vi "Lab Panel V4.90.vi"() -> ()   [LabVIEW 2013] (continued)
                              tunnel: [w5375 0] -> w5370
                              tunnel: w5371 -> [w5375 _]
                              tunnel: w5372 -> [_ w5376]
                              frame False {
                              }
                              frame True {
                                n2891 = Concatenate Strings("LA02-2 ", w5376) -> (w5379:string)
                                n2892 = One Button Dialog(message=w5379) -> ()  [unwired: 1 in, 1 out]
                              }
                            }
                          }
                          frame #4 {
                            n2893 = Greater?(x=w5381, y=w5384) -> (0:w5383:bool)
                            n2894 = case shown="True" w5383 {
                              tunnel: [w5385 0] -> w5380
                              tunnel: w5381 -> [w5385 _]
                              tunnel: w5382 -> [_ w5386]
                              frame False {
                              }
                              frame True {
                                n2895 = Concatenate Strings("LA03-1 ", w5386) -> (w5389:string)
                                n2896 = One Button Dialog(message=w5389) -> ()  [unwired: 1 in, 1 out]
                              }
                            }
                          }
                          frame #5 {
                            n2897 = Greater?(x=w5390, y=w5394) -> (0:w5393:bool)
                            n2898 = case shown="True" w5393 {
                              tunnel: [w5395 0] -> w5391
                              tunnel: w5390 -> [w5395 _]
                              tunnel: w5392 -> [_ w5396]
                              frame False {
                              }
                              frame True {
                                n2899 = Concatenate Strings("LA03-2 ", w5396) -> (w5399:string)
                                n2900 = One Button Dialog(message=w5399) -> ()  [unwired: 1 in, 1 out]
                              }
                            }
                          }
                          frame #6 {
                            n2901 = Greater?(x=w5401, y=w5404) -> (0:w5403:bool)
                            n2902 = case shown="True" w5403 {
                              tunnel: [w5405 0] -> w5400
                              tunnel: w5401 -> [w5405 _]
                              tunnel: w5402 -> [_ w5406]
                              frame False {
                              }
                              frame True {
                                n2903 = Concatenate Strings("LA04-1 ", w5406) -> (w5409:string)
                                n2904 = One Button Dialog(message=w5409) -> ()  [unwired: 1 in, 1 out]
                              }
                            }
                          }
                          frame #7 {
                            n2905 = Greater?(x=w5411, y=w5414) -> (0:w5413:bool)
                            n2906 = case shown="True" w5413 {
                              tunnel: [w5415 0] -> w5410
                              tunnel: w5411 -> [w5415 _]
                              tunnel: w5412 -> [_ w5416]
                              frame False {
                              }
                              frame True {
                                n2907 = Concatenate Strings("LA04-2 ", w5416) -> (w5419:string)
                                n2908 = One Button Dialog(message=w5419) -> ()  [unwired: 1 in, 1 out]
                              }
                            }
                          }
                          frame #8 {
                            n2909 = Greater?(x=w5421, y=w5424) -> (0:w5423:bool)
                            n2910 = case shown="True" w5423 {
                              tunnel: [w5425 0] -> w5420
                              tunnel: w5421 -> [w5425 _]
                              tunnel: w5422 -> [_ w5426]
                              frame False {
                              }
                              frame True {
                                n2911 = Concatenate Strings("LA05-1 ", w5426) -> (w5429:string)
                                n2912 = One Button Dialog(message=w5429) -> ()  [unwired: 1 in, 1 out]
                              }
                            }
                          }
                          frame #9 {
                            n2913 = Greater?(x=w5431, y=w5434) -> (0:w5433:bool)
                            n2914 = case shown="True" w5433 {
                              tunnel: [w5435 0] -> w5430
                              tunnel: w5431 -> [w5435 _]
                              tunnel: w5432 -> [_ w5436]
                              frame False {
                              }
                              frame True {
                                n2915 = Concatenate Strings("LA05-2 ", w5436) -> (w5439:string)
                                n2916 = One Button Dialog(message=w5439) -> ()  [unwired: 1 in, 1 out]
                              }
                            }
                          }
                        }
                        n2917 = Bundle By Name(cluster=w5338, "LAB01-1"=w5336, "LAB01-2"=w5334, "LAB02-1"=w5331, "LAB02-2"=w5328, "LAB03-1"=w5326, "LAB03-2"=w5325, "LAB04-1"=w5322, "LAB04-2"=w5320, "LAB05-1"=w5318, "LAB05-2"=w5316) -> (w5337:T8)
                        n2918 = local write "JIG RELAY CYCLES"(w5337) -> ()
                      }
                    }
                  }
                }
              }
            }
          }
          frame #19 {
            # "get temperature values"
            n2919 = local read "Panel #"() -> (w5440:dbl)
            n2920 = local read "simulate"() -> (w5453:bool)
            n2921 = local read "Temp Test Cal"() -> (w5450:dbl)
            n2922 = stacked-sequence {
              seq-local: [w5456 _] -> [_ w5492]
              tunnel: w5453 -> [_ w5506]
              tunnel: T14 {"1  (A) cal"=1.0, "1 (V) cal"=1.0, "1 (PF) cal"=1.0, "1 (TL) cal"=1.0, "1 (TN) cal"=1.0, "2 (A) cal"=1.0, "2 (V) cal"=1.0, "2 (PF) cal"=1.0, "2 (TL) cal"=1.0, "2 (TN) cal"=1.0} ("CAL LAB01") -> [_ w5505]
              tunnel: w5451 -> [_ w5504]
              tunnel: w5450 -> [_ w5503]
              tunnel: w5449 -> [_ w5502]
              tunnel: w5448 -> [_ w5501]
              tunnel: w5447 -> [_ w5500]
              tunnel: w5446 -> [_ w5499]
              tunnel: w5445 -> [_ w5498]
              tunnel: w5444 -> [_ w5497]
              tunnel: w5443 -> [_ w5496]
              tunnel: w5442 -> [_ w5495]
              tunnel: w5441 -> [_ w5494]
              tunnel: w5440 -> [_ w5493]
              frame #0 {
                n2923 = local read "Select COM port"() -> (w5457:refnum<visa-resource-name>)
                "COM port" <- w5457
                n2924 = global write "Global 1.vi" "COM port"(w5457) -> ()
                n2925 = global write "Global 1.vi" "tmp dly lps"("Temp Delay Lps") -> ()
                n2926 = global write "Global 1.vi" "dly value"("Temp Value") -> ()
                n2927 = local read "jig cycle"() -> (w5459:dbl)
                n2928 = local read "on loops"() -> (w5461:dbl)
                n2929 = Add(x=w5461, y=3) -> (x+y=w5462:dbl)
                n2930 = local read "Panel #"() -> (w5458:dbl)
                n2931 = Equal?(x=w5459, y=w5462) -> (x = y?=w5456:bool)
                n2932 = case shown="True" w5456 {
                  tunnel: w5458 -> [_ w5466]
                  frame False {
                  }
                  frame True {
                    n2933 = local read "simulate"() -> (w5463:bool)
                    n2934 = case shown="1" w5466 {
                      tunnel: 1.0 -> [_ w5471 w5473 w5479 w5483 w5488]
                      tunnel: w5463 -> [_ w5467 w5472 w5477 w5484 w5487]
                      frame 0, Default {
                      }
                      frame 1 {
                        w5469 = FALSE
                        n2935 = call "sub vi - GET ALL TEMP v6.vi"("LA01-EN"=TRUE, "simulate"=w5467, "LA02-EN"=w5469, "LA03-EN"=w5469, "LA04-EN"=w5469, "LA05-EN"=w5469, "Gen Cal Value"=w5471) -> ("LA01 TEMP"=w5468:T24)  [unwired: 3 in, 5 out]
                        n2936 = local write "LAB01 TEMP"(w5468) -> ()
                      }
                      frame 2 {
                        w5474 = FALSE
                        n2937 = call "sub vi - GET ALL TEMP v6.vi"("LA01-EN"=w5474, "simulate"=w5472, "LA02-EN"=TRUE, "LA03-EN"=w5474, "LA04-EN"=w5474, "LA05-EN"=w5474, "Gen Cal Value"=w5473) -> ("LA02 TEMP"=w5476:T24)  [unwired: 3 in, 5 out]
                        n2938 = local write "LAB02 TEMP"(w5476) -> ()
                      }
                      frame 3 {
                        w5480 = FALSE
                        n2939 = call "sub vi - GET ALL TEMP v6.vi"("LA01-EN"=w5480, "simulate"=w5477, "LA02-EN"=w5480, "LA03-EN"=TRUE, "LA04-EN"=w5480, "LA05-EN"=w5480, "Gen Cal Value"=w5479) -> ("LA03 TEMP"=w5478:T24)  [unwired: 3 in, 5 out]
                        n2940 = local write "LAB03 TEMP"(w5478) -> ()
                      }
                      frame 4 {
                        w5485 = FALSE
                        n2941 = call "sub vi - GET ALL TEMP v6.vi"("LA01-EN"=w5485, "simulate"=w5484, "LA02-EN"=w5485, "LA03-EN"=w5485, "LA04-EN"=TRUE, "LA05-EN"=w5485, "Gen Cal Value"=w5483) -> ("LA04 TEMP"=w5482:T24)  [unwired: 3 in, 5 out]
                        n2942 = local write "LAB04 TEMP"(w5482) -> ()
                      }
                      frame 5 {
                        w5490 = FALSE
                        n2943 = call "sub vi - GET ALL TEMP v6.vi"("LA01-EN"=w5490, "simulate"=w5487, "LA02-EN"=w5490, "LA03-EN"=w5490, "LA04-EN"=w5490, "LA05-EN"=TRUE, "Gen Cal Value"=w5488) -> ("LA05 TEMP"=w5489:T24)  [unwired: 3 in, 5 out]
                        n2944 = local write "LAB05 TEMP"(w5489) -> ()
                      }
                    }
                    n2945 = local write "TEMP"(TRUE) -> ()
                  }
                }
              }
              frame #1 {
                n2946 = case shown="True" w5492 {
                  tunnel: w5506 -> [_ w5520]
                  tunnel: w5505 -> [_ w5519]
                  tunnel: w5504 -> [_ w5518]
                  tunnel: w5503 -> [_ w5517]
                  tunnel: w5502 -> [_ w5516]
                  tunnel: w5501 -> [_ w5515]
                  tunnel: w5500 -> [_ w5514]
                  tunnel: w5499 -> [_ w5513]
                  tunnel: w5498 -> [_ w5512]
                  tunnel: w5497 -> [_ w5511]
                  tunnel: w5496 -> [_ w5510]
                  tunnel: w5495 -> [_ w5509]
                  tunnel: w5494 -> [_ w5508]
                  tunnel: w5493 -> [_ w5507]
                  frame False {
                  }
                  frame True {
                    n2947 = case shown="1" w5507 {
                      tunnel: w5520 -> [_ w5533 w5578 w5623 w5668 w5713]
                      tunnel: w5519 -> [_ w5532 w5577 w5622 w5667 w5712]
                      tunnel: w5518 -> [_ w5522 _ _ _ _]
                      tunnel: w5517 -> [_ w5527 w5576 w5621 w5666 w5711]
                      tunnel: w5516 -> [_ w5521 _ _ _ _]
                      tunnel: w5515 -> [_ _ w5567 _ _ _]
                      tunnel: w5514 -> [_ _ w5566 _ _ _]
                      tunnel: w5513 -> [_ _ _ w5612 _ _]
                      tunnel: w5512 -> [_ _ _ w5611 _ _]
                      tunnel: w5511 -> [_ _ _ _ w5657 _]
                      tunnel: w5510 -> [_ _ _ _ w5656 _]
                      tunnel: w5509 -> [_ _ _ _ _ w5702]
                      tunnel: w5508 -> [_ _ _ _ _ w5701]
                      frame ..0 {
                      }
                      frame 1 {
                        n2948 = case shown="False" w5533 {
                          tunnel: [w5564 w5565] -> w5549
                          tunnel: w5532 -> [_ w5565]
                          frame False {
                            n2949 = local read "CAL LAB01"() -> (w5564:T14)
                          }
                          frame True {
                          }
                        }
                        n2950 = local read "TEMP LA01"() -> (w5540:T9)
                        n2951 = local read "LAB01 TEMP"() -> (w5539:T12)
                        n2952 = call "sub vi - temperature delay v3.vi"("2-run"=w5521, "1-run"=w5522, "temp values IN"=w5540, "temp signals"=w5539) -> ("T2-N"=w5535:dbl, "T2-L"=w5536:dbl, "T1-N"=w5537:dbl, "T1-L"=w5538:dbl, "temp values OUT"=w5534:T43)  [unwired: 3 in]
                        n2953 = Unbundle By Name(w5549) -> ("1 (TL) cal"=w5544:dbl, "1 (TN) cal"=w5543:dbl, "2 (TL) cal"=w5542:dbl, "2 (TN) cal"=w5541:dbl)  [unwired: 6 out]
                        n2954 = local write "TEMP LA01"(w5534) -> ()
                        n2955 = Multiply(x=w5538, y=w5544) -> (x*y=w5531:dbl)
                        n2956 = Multiply(x=w5537, y=w5543) -> (x*y=w5529:dbl)
                        n2957 = Multiply(x=w5536, y=w5542) -> (x*y=w5526:dbl)
                        n2958 = Multiply(x=w5535, y=w5541) -> (x*y=w5525:dbl)
                        n2959 = case shown="True" w5522 {
                          tunnel: w5531 -> [w5558 w5563]
                          tunnel: w5527 -> [_ w5561]
                          tunnel: [w5558 w5562] -> w5530
                          tunnel: w5529 -> [w5557 w5560]
                          tunnel: [w5557 w5559] -> w5528
                          frame False {
                          }
                          frame True {
                            n2960 = Multiply(x=w5561, y=w5560) -> (x*y=w5559:dbl)
                            n2961 = Multiply(x=w5561, y=w5563) -> (x*y=w5562:dbl)
                          }
                        }
                        n2962 = case shown="True" w5521 {
                          tunnel: w5526 -> [w5551 w5556]
                          tunnel: w5527 -> [_ w5554]
                          tunnel: [w5551 w5555] -> w5524
                          tunnel: w5525 -> [w5550 w5553]
                          tunnel: [w5550 w5552] -> w5523
                          frame False {
                          }
                          frame True {
                            n2963 = Multiply(x=w5554, y=w5553) -> (x*y=w5552:dbl)
                            n2964 = Multiply(x=w5554, y=w5556) -> (x*y=w5555:dbl)
                          }
                        }
                        n2965 = local read "SIG LAB01-2"() -> (w5546:T2)
                        n2966 = local read "SIG LAB01-1"() -> (w5548:T2)
                        n2967 = Bundle By Name(cluster=w5548, "Tmp Live"=w5530, "Tmp Neut"=w5528) -> (w5547:T2)
                        n2968 = Bundle By Name(cluster=w5546, "Tmp Live"=w5524, "Tmp Neut"=w5523) -> (w5545:T2)
                        n2969 = local write "SIG LAB01-1"(w5547) -> ()
                        n2970 = local write "SIG LAB01-2"(w5545) -> ()
                      }
                      frame 2 {
                        n2971 = case shown="True" w5578 {
                          tunnel: [w5609 w5610] -> w5594
                          tunnel: w5577 -> [_ w5610]
                          frame False {
                            n2972 = local read "CAL LAB02"() -> (w5609:T15)
                          }
                          frame True {
                          }
                        }
                        n2973 = local read "LAB02 TEMP"() -> (w5585:T12)
                        n2974 = local read "TEMP LA02"() -> (w5584:T9)
                        n2975 = call "sub vi - temperature delay v3.vi"("2-run"=w5566, "1-run"=w5567, "temp values IN"=w5584, "temp signals"=w5585) -> ("T2-N"=w5579:dbl, "T2-L"=w5580:dbl, "T1-N"=w5581:dbl, "T1-L"=w5582:dbl, "temp values OUT"=w5583:T43)  [unwired: 3 in]
                        n2976 = Unbundle By Name(w5594) -> ("1 (TL) cal"=w5589:dbl, "1 (TN) cal"=w5588:dbl, "2 (TL) cal"=w5587:dbl, "2 (TN) cal"=w5586:dbl)  [unwired: 6 out]
                        n2977 = local write "TEMP LA02"(w5583) -> ()
                        n2978 = Multiply(x=w5582, y=w5589) -> (x*y=w5575:dbl)
                        n2979 = Multiply(x=w5581, y=w5588) -> (x*y=w5574:dbl)
                        n2980 = Multiply(x=w5580, y=w5587) -> (x*y=w5571:dbl)
                        n2981 = Multiply(x=w5579, y=w5586) -> (x*y=w5570:dbl)
                        n2982 = case shown="True" w5567 {
                          tunnel: w5575 -> [w5603 w5608]
                          tunnel: w5576 -> [_ w5606]
                          tunnel: [w5603 w5607] -> w5573
                          tunnel: w5574 -> [w5602 w5605]
                          tunnel: [w5602 w5604] -> w5572
                          frame False {
                          }
                          frame True {
                            n2983 = Multiply(x=w5606, y=w5605) -> (x*y=w5604:dbl)
                            n2984 = Multiply(x=w5606, y=w5608) -> (x*y=w5607:dbl)
                          }
                        }
                        n2985 = case shown="True" w5566 {
                          tunnel: w5571 -> [w5596 w5601]
                          tunnel: w5576 -> [_ w5599]
                          tunnel: [w5596 w5600] -> w5569
                          tunnel: w5570 -> [w5595 w5598]
                          tunnel: [w5595 w5597] -> w5568
                          frame False {
                          }
                          frame True {
                            n2986 = Multiply(x=w5599, y=w5598) -> (x*y=w5597:dbl)
                            n2987 = Multiply(x=w5599, y=w5601) -> (x*y=w5600:dbl)
                          }
                        }
                        n2988 = local read "SIG LAB02-2"() -> (w5591:T2)
                        n2989 = local read "SIG LAB02-1"() -> (w5593:T2)
                        n2990 = Bundle By Name(cluster=w5593, "Tmp Live"=w5573, "Tmp Neut"=w5572) -> (w5592:T2)
                        n2991 = Bundle By Name(cluster=w5591, "Tmp Live"=w5569, "Tmp Neut"=w5568) -> (w5590:T2)
                        n2992 = local write "SIG LAB02-1"(w5592) -> ()
                        n2993 = local write "SIG LAB02-2"(w5590) -> ()
                      }
                      frame 3 {
                        n2994 = case shown="False" w5623 {
                          tunnel: [w5654 w5655] -> w5639
                          tunnel: w5622 -> [_ w5655]
                          frame False {
                            n2995 = local read "CAL LAB03"() -> (w5654:T14)
                          }
                          frame True {
                          }
                        }
                        n2996 = local read "TEMP LA03"() -> (w5629:T9)
                        n2997 = local read "LAB03 TEMP"() -> (w5630:T12)
                        n2998 = call "sub vi - temperature delay v3.vi"("2-run"=w5611, "1-run"=w5612, "temp values IN"=w5629, "temp signals"=w5630) -> ("T2-N"=w5624:dbl, "T2-L"=w5625:dbl, "T1-N"=w5626:dbl, "T1-L"=w5627:dbl, "temp values OUT"=w5628:T43)  [unwired: 3 in]
                        n2999 = Unbundle By Name(w5639) -> ("1 (TL) cal"=w5634:dbl, "1 (TN) cal"=w5633:dbl, "2 (TL) cal"=w5632:dbl, "2 (TN) cal"=w5631:dbl)  [unwired: 6 out]
                        n3000 = local write "TEMP LA03"(w5628) -> ()
                        n3001 = Multiply(x=w5627, y=w5634) -> (x*y=w5620:dbl)
                        n3002 = Multiply(x=w5626, y=w5633) -> (x*y=w5619:dbl)
                        n3003 = Multiply(x=w5625, y=w5632) -> (x*y=w5616:dbl)
                        n3004 = Multiply(x=w5624, y=w5631) -> (x*y=w5615:dbl)
                        n3005 = case shown="True" w5611 {
                          tunnel: w5616 -> [w5641 w5646]
                          tunnel: w5621 -> [_ w5644]
                          tunnel: [w5641 w5645] -> w5614
                          tunnel: w5615 -> [w5640 w5643]
                          tunnel: [w5640 w5642] -> w5613
                          frame False {
                          }
                          frame True {
                            n3006 = Multiply(x=w5644, y=w5643) -> (x*y=w5642:dbl)
                            n3007 = Multiply(x=w5644, y=w5646) -> (x*y=w5645:dbl)
                          }
                        }
                        n3008 = case shown="True" w5612 {
                          tunnel: w5620 -> [w5648 w5653]
                          tunnel: w5621 -> [_ w5651]
                          tunnel: [w5648 w5652] -> w5618
                          tunnel: w5619 -> [w5647 w5650]
                          tunnel: [w5647 w5649] -> w5617
                          frame False {
                          }
                          frame True {
                            n3009 = Multiply(x=w5651, y=w5650) -> (x*y=w5649:dbl)
                            n3010 = Multiply(x=w5651, y=w5653) -> (x*y=w5652:dbl)
                          }
                        }
                        n3011 = local read "SIG LAB03-2"() -> (w5636:T2)
                        n3012 = local read "SIG LAB03-1"() -> (w5638:T2)
                        n3013 = Bundle By Name(cluster=w5638, "Tmp Live"=w5618, "Tmp Neut"=w5617) -> (w5637:T2)
                        n3014 = Bundle By Name(cluster=w5636, "Tmp Live"=w5614, "Tmp Neut"=w5613) -> (w5635:T2)
                        n3015 = local write "SIG LAB03-1"(w5637) -> ()
                        n3016 = local write "SIG LAB03-2"(w5635) -> ()
                      }
                      frame 4 {
                        n3017 = case shown="False" w5668 {
                          tunnel: [w5699 w5700] -> w5684
                          tunnel: w5667 -> [_ w5700]
                          frame False {
                            n3018 = local read "CAL LAB04"() -> (w5699:T14)
                          }
                          frame True {
                          }
                        }
                        n3019 = local read "LAB04 TEMP"() -> (w5674:T12)
                        n3020 = local read "TEMP LA04"() -> (w5675:T9)
                        n3021 = call "sub vi - temperature delay v3.vi"("2-run"=w5656, "1-run"=w5657, "temp values IN"=w5675, "temp signals"=w5674) -> ("T2-N"=w5669:dbl, "T2-L"=w5670:dbl, "T1-N"=w5671:dbl, "T1-L"=w5672:dbl, "temp values OUT"=w5673:T43)  [unwired: 3 in]
                        n3022 = Unbundle By Name(w5684) -> ("1 (TL) cal"=w5679:dbl, "1 (TN) cal"=w5678:dbl, "2 (TL) cal"=w5677:dbl, "2 (TN) cal"=w5676:dbl)  [unwired: 6 out]
                        n3023 = local write "TEMP LA04"(w5673) -> ()
                        n3024 = Multiply(x=w5672, y=w5679) -> (x*y=w5665:dbl)
                        n3025 = Multiply(x=w5671, y=w5678) -> (x*y=w5664:dbl)
                        n3026 = Multiply(x=w5670, y=w5677) -> (x*y=w5661:dbl)
                        n3027 = Multiply(x=w5669, y=w5676) -> (x*y=w5660:dbl)
                        n3028 = case shown="True" w5656 {
                          tunnel: w5661 -> [w5686 w5691]
                          tunnel: w5666 -> [_ w5689]
                          tunnel: [w5686 w5690] -> w5659
                          tunnel: w5660 -> [w5685 w5688]
                          tunnel: [w5685 w5687] -> w5658
                          frame False {
                          }
                          frame True {
                            n3029 = Multiply(x=w5689, y=w5688) -> (x*y=w5687:dbl)
                            n3030 = Multiply(x=w5689, y=w5691) -> (x*y=w5690:dbl)
                          }
                        }
                        n3031 = case shown="True" w5657 {
                          tunnel: w5665 -> [w5693 w5698]
                          tunnel: w5666 -> [_ w5696]
                          tunnel: [w5693 w5697] -> w5663
                          tunnel: w5664 -> [w5692 w5695]
                          tunnel: [w5692 w5694] -> w5662
                          frame False {
                          }
                          frame True {
                            n3032 = Multiply(x=w5696, y=w5695) -> (x*y=w5694:dbl)
                            n3033 = Multiply(x=w5696, y=w5698) -> (x*y=w5697:dbl)
                          }
                        }
                        n3034 = local read "SIG LAB04-2"() -> (w5681:T2)
                        n3035 = local read "SIG LAB04-1"() -> (w5683:T2)
                        n3036 = Bundle By Name(cluster=w5683, "Tmp Live"=w5663, "Tmp Neut"=w5662) -> (w5682:T2)
                        n3037 = Bundle By Name(cluster=w5681, "Tmp Live"=w5659, "Tmp Neut"=w5658) -> (w5680:T2)
                        n3038 = local write "SIG LAB04-1"(w5682) -> ()
                        n3039 = local write "SIG LAB04-2"(w5680) -> ()
                      }
                      frame 5.. {
                        n3040 = case shown="False" w5713 {
                          tunnel: [w5744 w5745] -> w5729
                          tunnel: w5712 -> [_ w5745]
                          frame False {
                            n3041 = local read "CAL LAB05"() -> (w5744:T14)
                          }
                          frame True {
                          }
                        }
                        n3042 = local read "LAB05 TEMP"() -> (w5719:T12)
                        n3043 = local read "TEMP LA05"() -> (w5720:T9)
                        n3044 = call "sub vi - temperature delay v3.vi"("2-run"=w5701, "1-run"=w5702, "temp values IN"=w5720, "temp signals"=w5719) -> ("T2-N"=w5715:dbl, "T2-L"=w5716:dbl, "T1-N"=w5717:dbl, "T1-L"=w5718:dbl, "temp values OUT"=w5714:T43)  [unwired: 3 in]
                        n3045 = local write "TEMP LA05"(w5714) -> ()
                        n3046 = Unbundle By Name(w5729) -> ("1 (TL) cal"=w5721:dbl, "1 (TN) cal"=w5724:dbl, "2 (TL) cal"=w5723:dbl, "2 (TN) cal"=w5722:dbl)  [unwired: 6 out]
                        n3047 = Multiply(x=w5718, y=w5721) -> (x*y=w5710:dbl)
                        n3048 = Multiply(x=w5717, y=w5724) -> (x*y=w5709:dbl)
                        n3049 = Multiply(x=w5716, y=w5723) -> (x*y=w5706:dbl)
                        n3050 = Multiply(x=w5715, y=w5722) -> (x*y=w5705:dbl)
                        n3051 = case shown="True" w5701 {
                          tunnel: w5706 -> [w5731 w5736]
                          tunnel: w5711 -> [_ w5734]
                          tunnel: [w5731 w5735] -> w5704
                          tunnel: w5705 -> [w5730 w5733]
                          tunnel: [w5730 w5732] -> w5703
                          frame False {
                          }
                          frame True {
                            n3052 = Multiply(x=w5734, y=w5733) -> (x*y=w5732:dbl)
                            n3053 = Multiply(x=w5734, y=w5736) -> (x*y=w5735:dbl)
                          }
                        }
                        n3054 = case shown="True" w5702 {
                          tunnel: w5710 -> [w5738 w5743]
                          tunnel: w5711 -> [_ w5741]
                          tunnel: [w5738 w5742] -> w5708
                          tunnel: w5709 -> [w5737 w5740]
                          tunnel: [w5737 w5739] -> w5707
                          frame False {
                          }
                          frame True {
                            n3055 = Multiply(x=w5741, y=w5740) -> (x*y=w5739:dbl)
                            n3056 = Multiply(x=w5741, y=w5743) -> (x*y=w5742:dbl)
                          }
                        }
                        n3057 = local read "SIG LAB05-1"() -> (w5728:T2)
                        n3058 = Bundle By Name(cluster=w5728, "Tmp Live"=w5708, "Tmp Neut"=w5707) -> (w5727:T2)
                        n3059 = local read "SIG LAB05-2"() -> (w5726:T2)
                        n3060 = Bundle By Name(cluster=w5726, "Tmp Live"=w5704, "Tmp Neut"=w5703) -> (w5725:T2)
                        n3061 = local write "SIG LAB05-1"(w5727) -> ()
                        n3062 = local write "SIG LAB05-2"(w5725) -> ()
                      }
                    }
                  }
                }
              }
            }
          }
          frame #20 {
            # "write data to display panel"
            n3063 = global write "Global display 1.vi" "TEST 5-2"(w5780) -> ()
            n3064 = global write "Global display 1.vi" "TEST 4-2"(w5782) -> ()
            n3065 = global write "Global display 1.vi" "TEST 1-2"(w5788) -> ()
            n3066 = global write "Global display 1.vi" "TEST 3-1"(w5785) -> ()
            n3067 = global write "Global display 1.vi" "TEST 5-1"(w5781) -> ()
            n3068 = global write "Global display 1.vi" "TEST 1-1"(w5789) -> ()
            n3069 = global write "Global display 1.vi" "TEST 3-2"(w5784) -> ()
            n3070 = global write "Global display 1.vi" "TEST 4-1"(w5783) -> ()
            n3071 = global write "Global display 1.vi" "TEST 2-2"(w5786) -> ()
            n3072 = global write "Global display 1.vi" "TEST 2-1"(w5787) -> ()
            n3073 = global read "Global display 3.vi" "log 1-1"() -> (→"LOG LAB01-1":string)
            n3074 = global read "Global display 3.vi" "log 3-1"() -> (→"LOG LAB03-1":string)
            n3075 = global read "Global display 3.vi" "log 1-2"() -> (→"LOG LAB01-2":string)
            n3076 = property on="Tab Control 2" class="TabCtl (strict)"() -> ("Pages"=w5779:refnum<vi>[])  [unwired: 2 in, 2 out]
            n3077 = global read "Global display 3.vi" "log 2-1"() -> (→"LOG LAB02-1":string)
            n3078 = global read "Global display 3.vi" "log 2-2"() -> (→"LOG LAB02-2":string)
            n3079 = global read "Global display 3.vi" "log 4-2"() -> (→"LOG LAB04-2":string)
            n3080 = global read "Global display 3.vi" "log 5-2"() -> (→"LOG LAB05-2":string)
            n3081 = global read "Global display 3.vi" "log 5-1"() -> (→"LOG LAB05-1":string)
            n3082 = global read "Global display 3.vi" "log 4-1"() -> (→"LOG LAB04-1":string)
            n3083 = global read "Global display 3.vi" "log 3-2"() -> (→"LOG LAB03-2":string)
            n3084 = Index Array(array=w5779, index=8) -> (element=w5777:refnum<vi>)
            n3085 = property class="Page"(reference=w5777) -> ("PageVis"=w5776:bool)  [unwired: 1 in, 2 out]
            n3086 = global write "Global display 3.vi" "admin"(w5776) -> ()
            n3087 = local read "O/I  LAB05-2"() -> (w5830:bool)
            n3088 = local read "O/I  LAB05-1"() -> (w5831:bool)
            n3089 = local read "O/I  LAB03-2"() -> (w5834:bool)
            n3090 = local read "O/I  LAB04-2"() -> (w5832:bool)
            n3091 = local read "O/I  LAB04-1"() -> (w5833:bool)
            n3092 = local read "O/I  LAB03-1"() -> (w5835:bool)
            n3093 = local read "O/I  LAB01-2"() -> (w5838:bool)
            n3094 = local read "O/I  LAB01-1"() -> (w5839:bool)
            n3095 = local read "O/I  LAB02-1"() -> (w5837:bool)
            n3096 = local read "O/I  LAB02-2"() -> (w5836:bool)
            n3097 = global write "Global display 1.vi" "5-2 O/F"(w5830) -> ()
            n3098 = global write "Global display 1.vi" "5-1 O/F"(w5831) -> ()
            n3099 = global write "Global display 1.vi" "4-1 O/F"(w5833) -> ()
            n3100 = global write "Global display 1.vi" "4-2 O/F"(w5832) -> ()
            n3101 = global write "Global display 1.vi" "3-2 O/F"(w5834) -> ()
            n3102 = global write "Global display 1.vi" "3-1 O/F"(w5835) -> ()
            n3103 = global write "Global display 1.vi" "2-2 O/F"(w5836) -> ()
            n3104 = global write "Global display 1.vi" "2-1 O/F"(w5837) -> ()
            n3105 = global write "Global display 1.vi" "1-2 O/F"(w5838) -> ()
            n3106 = global write "Global display 1.vi" "1-1 O/F"(w5839) -> ()
            n3107 = local read "TEMP START LAB02-2"() -> (w5762:cluster{"TL":dbl, "TN":dbl})
            n3108 = local read "run lab05-2"() -> (w5820:bool)
            n3109 = local read "TEMP START LAB01-2"() -> (w5764:cluster{"TL":dbl, "TN":dbl})
            n3110 = local read "TEMP START LAB02-1"() -> (w5763:cluster{"TL":dbl, "TN":dbl})
            n3111 = local read "TEMP START LAB04-1"() -> (w5759:cluster{"TL":dbl, "TN":dbl})
            n3112 = local read "TEMP START LAB04-2"() -> (w5758:cluster{"TL":dbl, "TN":dbl})
            n3113 = local read "run lab04-1"() -> (w5823:bool)
            n3114 = local read "run lab04-2"() -> (w5822:bool)
            n3115 = local read "run lab05-1"() -> (w5821:bool)
            n3116 = local read "TEMP START LAB01-1"() -> (w5765:cluster{"TL":dbl, "TN":dbl})
            n3117 = local read "TEMP START LAB05-2"() -> (w5756:cluster{"TL":dbl, "TN":dbl})
            n3118 = local read "TEMP START LAB05-1"() -> (w5757:cluster{"TL":dbl, "TN":dbl})
            n3119 = local read "run lab03-2"() -> (w5824:bool)
            n3120 = local read "TEMP START LAB03-2"() -> (w5760:cluster{"TL":dbl, "TN":dbl})
            n3121 = local read "TEMP START LAB03-1"() -> (w5761:cluster{"TL":dbl, "TN":dbl})
            n3122 = local read "run lab02-1"() -> (w5827:bool)
            n3123 = local read "run lab03-1"() -> (w5825:bool)
            n3124 = local read "run lab01-2"() -> (w5828:bool)
            n3125 = local read "run lab02-2"() -> (w5826:bool)
            n3126 = local read "run lab01-1"() -> (w5829:bool)
            n3127 = global write "Global display 1.vi" "5-2 R/S"(w5820) -> ()
            n3128 = global write "Global display 1.vi" "5-1 R/S"(w5821) -> ()
            n3129 = global write "Global display 1.vi" "4-2 R/S"(w5822) -> ()
            n3130 = global write "Global display 1.vi" "4-1 R/S"(w5823) -> ()
            n3131 = global write "Global display 1.vi" "3-2 R/S"(w5824) -> ()
            n3132 = global write "Global display 1.vi" "1-2 R/S"(w5828) -> ()
            n3133 = global write "Global display 1.vi" "2-1 R/S"(w5827) -> ()
            n3134 = global write "Global display 1.vi" "3-1 R/S"(w5825) -> ()
            n3135 = global write "Global display 1.vi" "2-2 R/S"(w5826) -> ()
            n3136 = global write "Global display 1.vi" "1-1 R/S"(w5829) -> ()
            n3137 = global write "Global display 3.vi" "TEMP ST 05-2"(w5756) -> ()
            n3138 = global write "Global display 3.vi" "TEMP ST 05-1"(w5757) -> ()
            n3139 = global write "Global display 3.vi" "TEMP ST 03-2"(w5760) -> ()
            n3140 = global write "Global display 3.vi" "TEMP ST 04-2"(w5758) -> ()
            n3141 = global write "Global display 3.vi" "TEMP ST 01-1"(w5765) -> ()
            n3142 = global write "Global display 3.vi" "TEMP ST 01-2"(w5764) -> ()
            n3143 = global write "Global display 3.vi" "TEMP ST 04-1"(w5759) -> ()
            n3144 = global write "Global display 3.vi" "TEMP ST 02-1"(w5763) -> ()
            n3145 = global write "Global display 3.vi" "TEMP ST 02-2"(w5762) -> ()
            n3146 = global write "Global display 3.vi" "TEMP ST 03-1"(w5761) -> ()
            n3147 = local read "DISP LAB04-2"() -> (w5812:T4)
            n3148 = local read "DISP LAB05-1"() -> (w5811:T4)
            n3149 = local read "DISP LAB04-1"() -> (w5813:T4)
            n3150 = local read "DISP LAB05-2"() -> (w5810:T4)
            n3151 = local read "DISP LAB03-1"() -> (w5815:T4)
            n3152 = local read "DISP LAB03-2"() -> (w5814:T4)
            n3153 = local read "DISP LAB01-2"() -> (w5818:T4)
            n3154 = local read "DISP LAB02-1"() -> (w5817:T4)
            n3155 = local read "DISP LAB02-2"() -> (w5816:T4)
            n3156 = local read "DISP LAB01-1"() -> (w5819:T4)
            n3157 = local read "TEMP RISE LAB05-1"() -> (w5747:cluster{"TL":dbl, "TN":dbl})
            n3158 = local read "TEMP RISE LAB05-2"() -> (w5746:cluster{"TL":dbl, "TN":dbl})
            n3159 = local read "TEMP RISE LAB04-2"() -> (w5748:cluster{"TL":dbl, "TN":dbl})
            n3160 = local read "TEMP RISE LAB04-1"() -> (w5749:cluster{"TL":dbl, "TN":dbl})
            n3161 = local read "TEMP RISE LAB03-2"() -> (w5750:cluster{"TL":dbl, "TN":dbl})
            n3162 = local read "TEMP RISE LAB03-1"() -> (w5751:cluster{"TL":dbl, "TN":dbl})
            n3163 = local read "TEMP RISE LAB01-2"() -> (w5754:cluster{"TL":dbl, "TN":dbl})
            n3164 = local read "TEMP RISE LAB02-2"() -> (w5752:cluster{"TL":dbl, "TN":dbl})
            n3165 = local read "TEMP RISE LAB01-1"() -> (w5755:cluster{"TL":dbl, "TN":dbl})
            n3166 = local read "TEMP RISE LAB02-1"() -> (w5753:cluster{"TL":dbl, "TN":dbl})
            n3167 = global write "Global display 2.vi" "DISP LAB05-1"(w5811) -> ()
            n3168 = global write "Global display 2.vi" "DISP LAB05-2"(w5810) -> ()
            n3169 = global write "Global display 2.vi" "DISP LAB04-2"(w5812) -> ()
            n3170 = global write "Global display 2.vi" "DISP LAB02-1"(w5817) -> ()
            n3171 = global write "Global display 2.vi" "DISP LAB02-2"(w5816) -> ()
            n3172 = global write "Global display 2.vi" "DISP LAB04-1"(w5813) -> ()
            n3173 = global write "Global display 2.vi" "DISP LAB01-2"(w5818) -> ()
            n3174 = global write "Global display 2.vi" "DISP LAB01-1"(w5819) -> ()
            n3175 = global write "Global display 2.vi" "DISP LAB03-1"(w5815) -> ()
            n3176 = global write "Global display 2.vi" "DISP LAB03-2"(w5814) -> ()
            n3177 = global write "Global display 3.vi" "TEMP RS 05-2"(w5746) -> ()
            n3178 = global write "Global display 3.vi" "TEMP RS 05-1"(w5747) -> ()
            n3179 = global write "Global display 3.vi" "TEMP RS 03-2"(w5750) -> ()
            n3180 = global write "Global display 3.vi" "TEMP RS 02-1"(w5753) -> ()
            n3181 = global write "Global display 3.vi" "TEMP RS 02-2"(w5752) -> ()
            n3182 = global write "Global display 3.vi" "TEMP RS 04-2"(w5748) -> ()
            n3183 = global write "Global display 3.vi" "TEMP RS 01-2"(w5754) -> ()
            n3184 = global write "Global display 3.vi" "TEMP RS 03-1"(w5751) -> ()
            n3185 = global write "Global display 3.vi" "TEMP RS 04-1"(w5749) -> ()
            n3186 = global write "Global display 3.vi" "TEMP RS 01-1"(w5755) -> ()
            n3187 = local read "SET LAB05-2"() -> (w5800:T5)
            n3188 = local read "SET LAB05-1"() -> (w5801:T5)
            n3189 = local read "SET LAB04-1"() -> (w5803:T5)
            n3190 = local read "SET LAB04-2"() -> (w5802:T5)
            n3191 = local read "SET LAB03-1"() -> (w5805:T5)
            n3192 = local read "SET LAB03-2"() -> (w5804:T5)
            n3193 = local read "SET LAB02-2"() -> (w5806:T5)
            n3194 = local read "SET LAB01-2"() -> (w5808:T5)
            n3195 = local read "SET LAB02-1"() -> (w5807:T5)
            n3196 = local read "SET LAB01-1"() -> (w5809:T5)
            n3197 = global write "Global display 2.vi" "SET LAB05-2"(w5800) -> ()
            n3198 = global write "Global display 2.vi" "SET LAB05-1"(w5801) -> ()
            n3199 = global write "Global display 2.vi" "SET LAB04-1"(w5803) -> ()
            n3200 = global write "Global display 2.vi" "SET LAB04-2"(w5802) -> ()
            n3201 = global write "Global display 2.vi" "SET LAB03-2"(w5804) -> ()
            n3202 = global write "Global display 2.vi" "SET LAB02-2"(w5806) -> ()
            n3203 = global write "Global display 2.vi" "SET LAB03-1"(w5805) -> ()
            n3204 = global write "Global display 2.vi" "SET LAB01-2"(w5808) -> ()
            n3205 = global write "Global display 2.vi" "SET LAB01-1"(w5809) -> ()
            n3206 = global write "Global display 2.vi" "SET LAB02-1"(w5807) -> ()
            n3207 = local read "RESULT LAB01-1"() -> (w5799:bool)
            n3208 = local read "RESULT LAB03-2"() -> (w5794:bool)
            n3209 = local read "RESULT LAB04-1"() -> (w5793:bool)
            n3210 = local read "RESULT LAB04-2"() -> (w5792:bool)
            n3211 = local read "RESULT LAB02-2"() -> (w5796:bool)
            n3212 = local read "RESULT LAB01-2"() -> (w5798:bool)
            n3213 = local read "RESULT LAB02-1"() -> (w5797:bool)
            n3214 = local read "RESULT LAB03-1"() -> (w5795:bool)
            n3215 = local read "RESULT LAB05-1"() -> (w5791:bool)
            n3216 = local read "RESULT LAB05-2"() -> (w5790:bool)
            n3217 = global write "Global display 2.vi" "RESULT LAB05-1"(w5791) -> ()
            n3218 = global write "Global display 2.vi" "RESULT LAB01-2"(w5798) -> ()
            n3219 = global write "Global display 2.vi" "RESULT LAB03-2"(w5794) -> ()
            n3220 = global write "Global display 2.vi" "RESULT LAB04-1"(w5793) -> ()
            n3221 = global write "Global display 2.vi" "RESULT LAB04-2"(w5792) -> ()
            n3222 = global write "Global display 2.vi" "RESULT LAB05-2"(w5790) -> ()
            n3223 = global write "Global display 2.vi" "RESULT LAB03-1"(w5795) -> ()
            n3224 = global write "Global display 2.vi" "RESULT LAB02-1"(w5797) -> ()
            n3225 = global write "Global display 2.vi" "RESULT LAB02-2"(w5796) -> ()
            n3226 = global write "Global display 2.vi" "RESULT LAB01-1"(w5799) -> ()
          }
          frame #21 {
            # "simulate values"
            n3227 = global write "Global display 4.vi" "LAB deg C"("LAB deg C") -> ()
          }
          frame #22 {
            # "end main and display program"
            n3228 = Quit LabVIEW(quit? (T)="stop all") -> ()
            n3229 = global write "Global display 1.vi" "stop disp"("stop all") -> ()
          }
        }
        n3230 = node-c288() -> ()  [unwired: 1 in, 1 out]
        "loops" <- w309
      }
      n3231 = node-c288(w286) -> ()  [unwired: 1 out]
    }
  }
